vi "Export time-lapse subset-path management.vi"(11 "AVI path in":path) -> (1 "cancelled":bool, 2 "New folder path":path, 3 "Existing AVI path":path)   [LabVIEW 2013]
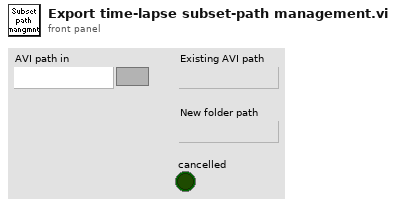
[diagram p1: front panel]
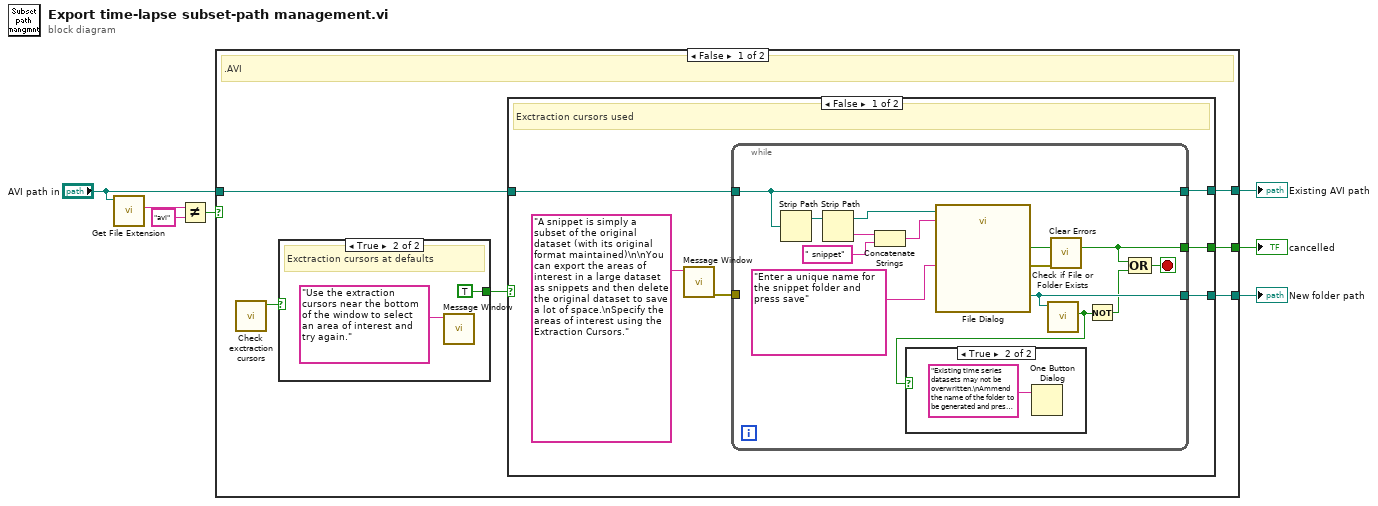
[diagram p0: block diagram]
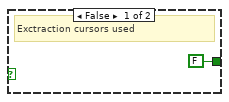
[diagram p2: hidden frame]
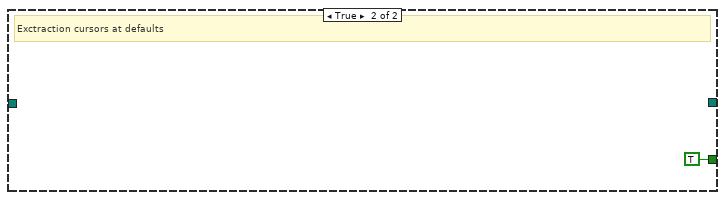
[diagram p4: hidden frame]
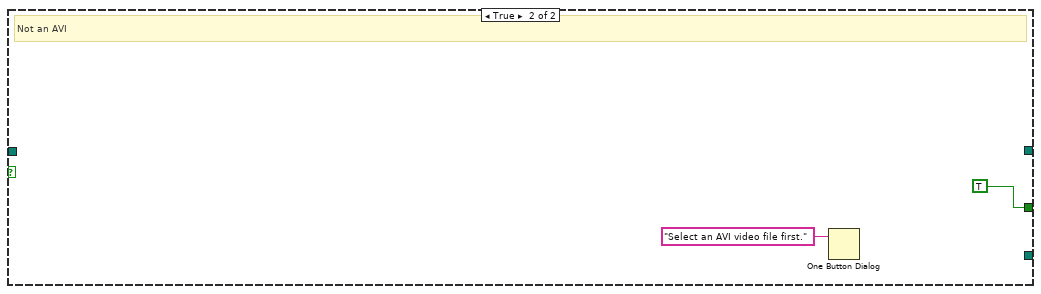
[diagram p5: hidden frame]
diagram:
  n1 = call <vilib>:"Get File Extension.vi"("file"="AVI path in") -> ("lowercase file extension"=w2:string)  [unwired: 7 in, 3 out]
  n2 = Not Equal?(x=w2, y="avi") -> (x != y?=w4:bool)
  n3 = case shown="False" w4 {
    tunnel: [w10 _] -> w6
    tunnel: [w13 TRUE ("cancelled")] -> w5
    tunnel: "AVI path in" -> [w12 _]
    tunnel: [w11 _] -> w7
    frame False {
      # ".AVI"
      n4 = call "Check exctraction cursors.vi"() -> ("Extraction cursors at default positions"=w9:bool)  [unwired: 9 in, 2 out]
      n5 = case shown="True" w9 {
        tunnel: [FALSE TRUE] -> w8
        frame False {
          # "Exctraction cursors used"
        }
        frame True {
          # "Exctraction cursors at defaults"
          n6 = call "Message Window.vi"("Message string"="Use the extraction cursors near the bottom of the window to select an area of interest and try again.") -> ()  [unwired: 10 in, 1 out]
        }
      }
      n7 = case shown="False" w8 {
        tunnel: [w22 TRUE ("cancelled")] -> w13
        tunnel: w12 -> [w21 _]
        tunnel: [w20 _] -> w11
        tunnel: [w19 _] -> w10
        frame False {
          # "Exctraction cursors used"
          n8 = call "Message Window.vi"("Message string"="A snippet is simply a subset of the original dataset (with its original format maintained)\n\nYou can export the areas of interest in a large dataset as snippets and then delete the original dataset to save a lot of space.\nSpecify the areas of interest using the Extraction Cursors.") -> ("error out (no error)"=w17:errorcluster)  [unwired: 10 in]
          n9 = while {
            tunnel: [w28] -> w22
            tunnel: w21 -> [w29]
            tunnel: [w26] -> w20
            tunnel: [w29] -> w19
            tunnel: w17 -> [_]
            stop <- w27 stop-if-true
            n10 = Strip Path(path=w29) -> (stripped path=w35:path)  [unwired: 1 out]
            n11 = Strip Path(path=w35) -> (stripped path=w32:path, name=w34:string)
            n12 = Concatenate Strings(w34, " snippet" ("format string")) -> (w30:string)
            n13 = call "File Dialog"("start path"=w32, "prompt"="Enter a unique name for the snippet folder and press save", "default name"=w30) -> ("selected path"=w26:path, "cancelled"=w28:bool, "error out"=w31:errorcluster)  [unwired: 9 in, 1 out]
            n14 = call <vilib>:"Check if File or Folder Exists.vi"("path"=w26) -> ("file or folder exists?"=w23:bool)  [unwired: 8 in, 2 out]
            n15 = case shown="True" w23 {
              frame False {
              }
              frame True {
                n16 = One Button Dialog(message="Existing time series datasets may not be overwritten.\nAmmend the name of the folder to be generated and press Save.") -> ()  [unwired: 1 in, 1 out]
              }
            }
            n17 = call <vilib>:"Clear Errors.vi"("error in (no error)"=w31) -> ()  [unwired: 6 in, 1 out]
            n18 = Not(x=w23) -> (.not. x?=w25:bool)
            n19 = Compound Arithmetic op=OR(w28, w25) -> (w27:bool)
          }
        }
        frame True {
          # "Exctraction cursors at defaults"
        }
      }
    }
    frame True {
      # "Not an AVI"
      n20 = One Button Dialog(message="Select an AVI video file first.") -> ()  [unwired: 1 in, 1 out]
    }
  }
  "New folder path" <- w7
  "Existing AVI path" <- w6
  "cancelled" <- w5
